vi "General Pulse Train.vi"(7 "prototype spec":T1={"Prototype Pulse"=[], "delta t of Prototype Pulse"=0.1}, 8 "method":i32(ring)=1 items=["nearest", "linear", "spline", "cubic Hermite"], 9 "Delay":dbl[](array[numeric]), 10 "Amplitude":dbl[](array[numeric]), 11 "X":dbl[](array[numeric])) -> (0 "error":i32, 3 "Pulse Train":dbl[](array[numeric]))   [LabVIEW 2017, in "NI_AALBase.lvlib"]
uses:
  <vilib>/Analysis/NI_AALBase.lvlib
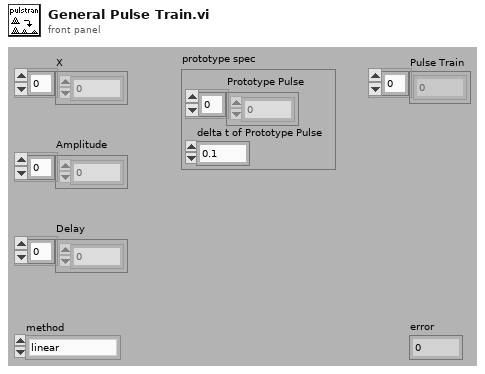
[diagram p1: front panel]
types:
  T1 = cluster{"Prototype Pulse":dbl[], "delta t of Prototype Pulse":dbl}
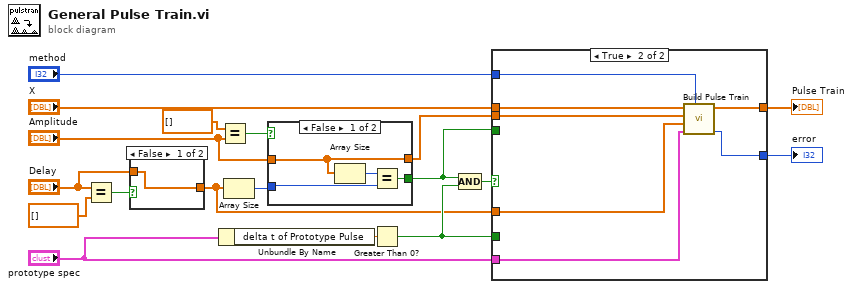
[diagram p0: block diagram]
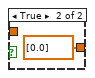
[diagram p2: hidden frame]
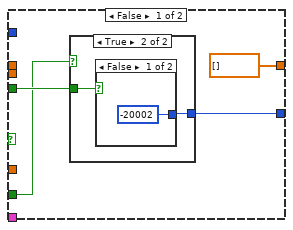
[diagram p3: hidden frame]
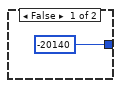
[diagram p4: hidden frame]
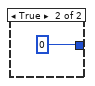
[diagram p5: hidden frame]
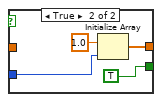
[diagram p6: hidden frame]
diagram:
  n1 = Equal?(x="Delay", y=dbl[] []) -> (x = y?=w4:bool)
  n2 = case shown="False" w4 {
    tunnel: [w19 dbl[] [0.0]] -> w8
    tunnel: "Delay" -> [w19 _]
    frame False {
    }
    frame True {
    }
  }
  n3 = Unbundle By Name("prototype spec") -> ("delta t of Prototype Pulse"=w16:dbl)
  n4 = Equal?(x=dbl[] [], y="Amplitude") -> (x = y?=w1:bool)
  n5 = Array Size(array=w8) -> (size(s)=w18:i32)
  n6 = case shown="False" w1 {
    tunnel: w18 -> [w21 w28]
    tunnel: [w24 w26] -> w9
    tunnel: [w23 TRUE] -> w15
    tunnel: "Amplitude" -> [w24 _]
    frame False {
      n7 = Array Size(array=w24) -> (size(s)=w22:i32)
      n8 = Equal?(x=w22, y=w21) -> (x = y?=w23:bool)
    }
    frame True {
      n9 = Initialize Array(1.0 ("element"), w28) -> (w26:dbl[])
    }
  }
  n10 = Greater Than 0?(x=w16) -> (x > 0?=w14:bool)
  n11 = Compound Arithmetic op=AND(w15, w14) -> (w17:bool)
  n12 = case shown="True" w17 {
    tunnel: w15 -> [w30 _]
    tunnel: w14 -> [w29 _]
    tunnel: "prototype spec" -> [_ w44]
    tunnel: w9 -> [_ w43]
    tunnel: w8 -> [_ w42]
    tunnel: "method" -> [_ w41]
    tunnel: [dbl[] [] w40] -> w10
    tunnel: [w31 w39] -> w11
    tunnel: "X" -> [_ w38]
    frame False {
      n13 = case shown="True" w29 {
        tunnel: [-20140 w34] -> w31
        tunnel: w30 -> [_ w35]
        frame False {
        }
        frame True {
          n14 = case shown="False" w35 {
            tunnel: [-20002 0] -> w34
            frame False {
            }
            frame True {
            }
          }
        }
      }
    }
    frame True {
      n15 = call <vilib>:"Build Pulse Train.vi"("method"=w41, "prototype spec"=w44, "Delay"=w42, "Amplitude"=w43, "X"=w38) -> ("error"=w39:i32, "Pulse Train"=w40:dbl[])  [unwired: 5 in]
    }
  }
  "error" <- w11
  "Pulse Train" <- w10
